vi "scope_amp.vi"(10 "error in (no error)":errorcluster, 11 "VISA resource name":refnum<visa-resource-name>) -> (0 "Waveform Data":waveform(dbl)(graph), 1 "error out":errorcluster, 2 "detected amplitude":dbl format="%.2p", 3 "detected frequency":dbl format="%.2p")   [LabVIEW 2015]
uses:
  <instrlib>/Tektronix TDS 200 1000 2000 Series/Public/Data/Read (Single Waveform).vi
  <vilib>/measure/matone.llb/Extract Single Tone Information 1 Chan.vi
  <vilib>/measure/NI_MAPro.lvlib
  <instrlib>/Tektronix TDS 200 1000 2000 Series/Tektronix TDS 200 1000 2000 Series.lvlib
panel:
  out "VISA resource name out":refnum<visa-resource-name>
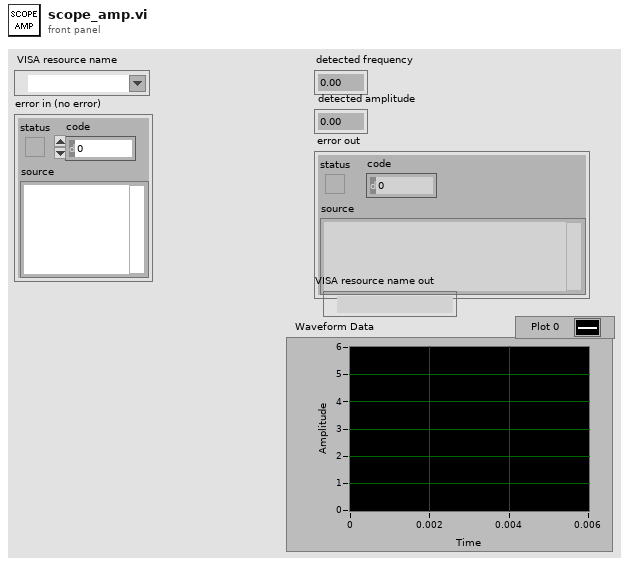
[diagram p1: front panel]
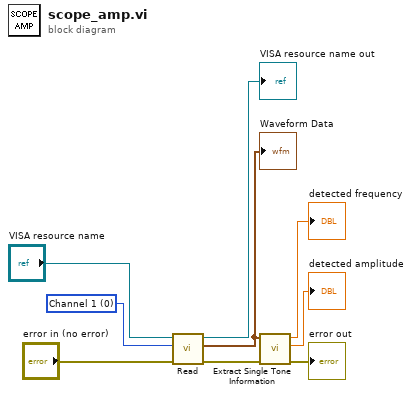
[diagram p0: block diagram]
diagram:
  w5 = u16 0 items=["Channel 1", "Channel 2", "Channel 3", "Channel 4", "Math", "Reference A", "Reference B", "Reference C", "Reference D", "FFT"] ("Source (0: Channel 1)")
  n1 = call-poly <instrlib>:"Read.vi"("error in (no error)"="error in (no error)", "Source (0: Channel 1)"=w5, "VISA resource name"="VISA resource name") -> ("error out"=w1:errorcluster, "Waveform Data"=w3:waveform(dbl), "VISA resource name out"=→"VISA resource name out":refnum<visa-resource-name>)  [unwired: 6 in]
  "Waveform Data" <- w3
  n2 = call-poly <vilib>:"Extract Single Tone Information.vi"("error in (no error)"=w1, "time signal in"=w3) -> ("error out"=→"error out":errorcluster, "detected amplitude"=→"detected amplitude":dbl, "detected frequency"=→"detected frequency":dbl)  [unwired: 4 in, 3 out]
